vi "Continue Cycle Test.vi"(8 "error in (no error)":errorcluster, 11 "Controller in":refnum<class "Controller.lvclass">) -> (0 "error out":errorcluster, 2 "Status String":string, 3 "Controller out":refnum<class "Controller.lvclass">)   [LabVIEW 2020, in "Controller.lvlib" / "Controller.lvclass"]
uses:
  Controller.lvclass
  Controller.lvclass/Controller.ctl
  Actor_AFG/Actor_AFG Messages/AFG Wait for Complete Msg/AFG Wait for Complete Msg.lvclass/AFG Wait for Complete Msg.ctl
  <vilib>/ActorFramework/Message Enqueuer/Message Enqueuer.lvclass/Message Enqueuer.ctl
  Main_UI/Main_UI Messages/Update Cycle States Msg/Update Cycle States Msg.lvclass/Update Cycle States Msg.ctl
  <vilib>/ActorFramework/Message Enqueuer/Enqueue.vi
  Actor_AFG/Actor_AFG Messages/AFG Wait for Complete Msg/AFG Wait for Complete Msg.lvclass
  C:/Program Files/National Instruments/LabVIEW 2020/vi.lib/ActorFramework/Message/Message.lvclass
  Main_UI/Main_UI Messages/Update Cycle States Msg/Update Cycle States Msg.lvclass
  <vilib>/ActorFramework/Message Priority Queue/Priority Enqueue.vi
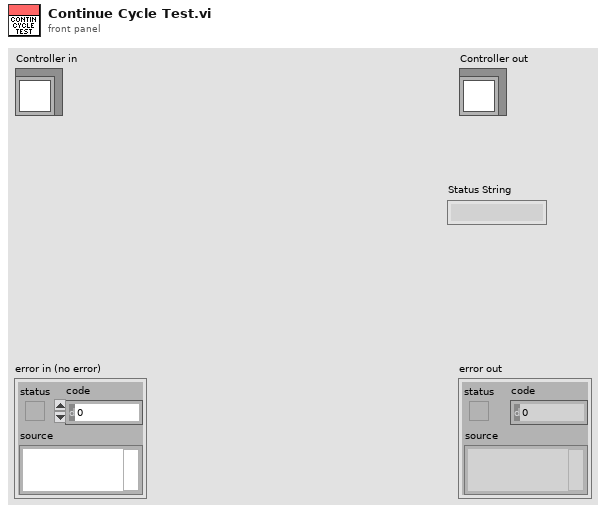
[diagram p1: front panel]
types:
  T1 = enum16{"Single Pulse", "Cycle_Idle", "Cycle_Running", "Cycle_Pause"}
  T2 = cluster{"Set Pulse Conf":cluster{"V Conf":cluster{"Bias":dbl, "Amp":dbl}, "T Conf":cluster{"Rise Time":dbl, "Fall Time":dbl, "Pulse Width":dbl}}, "Reset Pulse Conf":cluster{"V Conf":cluster{"Bias":dbl, "Amp":dbl}, "T Conf":cluster{"Rise Time":dbl, "Fall Time":dbl, "Pulse Width":dbl}}, "Cycle Timing":cluster{"Delay":dbl, "Pulse Spacing":dbl, "Burst Counts:":dbl, "Read Counts:":dbl}, "Read Voltage Setting":dbl}
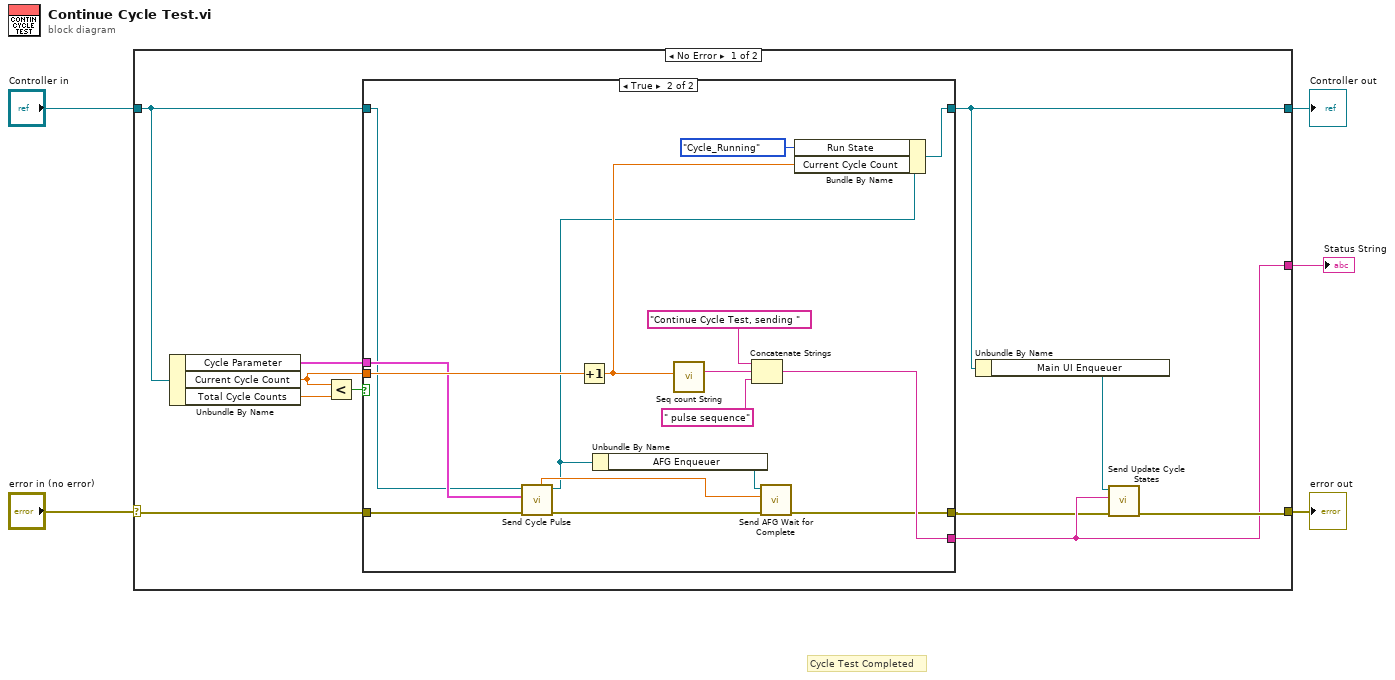
[diagram p0: block diagram]
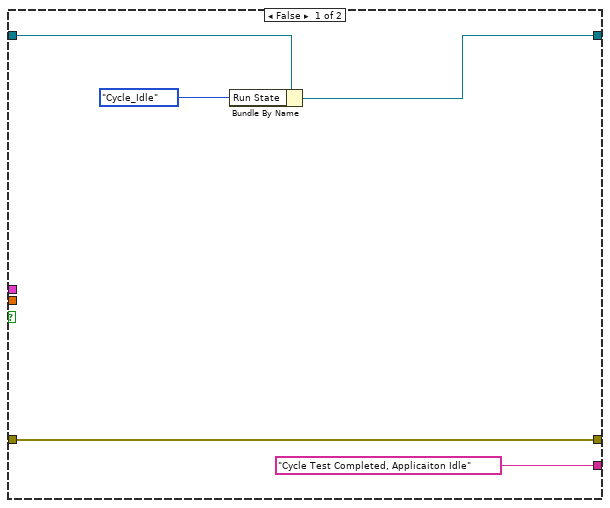
[diagram p2: hidden frame]
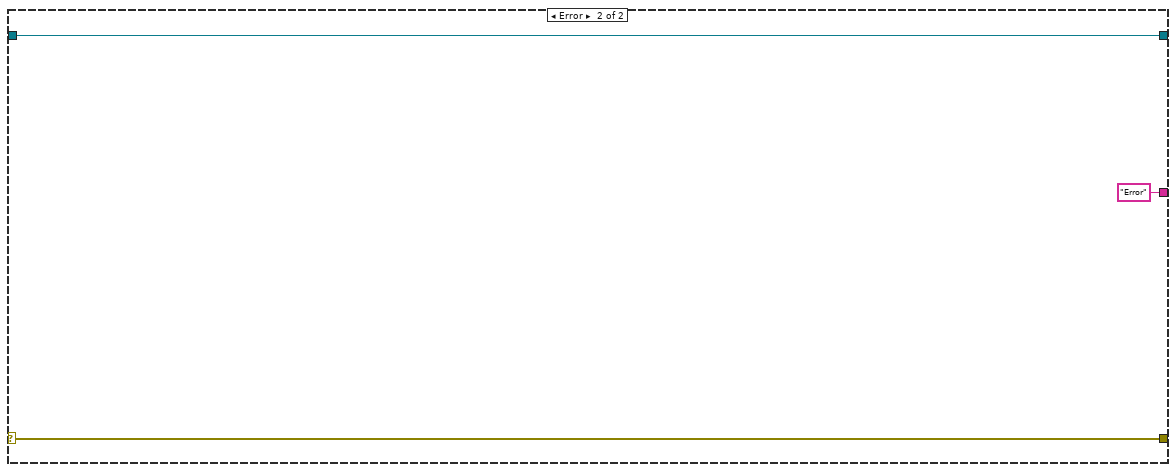
[diagram p3: hidden frame]
diagram:
  # "Cycle Test Completed"
  n1 = case shown="No Error" "error in (no error)" {
    selector: "error in (no error)" -> [w13 w40]
    tunnel: [w9 w40] -> w4
    tunnel: [w10 w39] -> w2
    tunnel: "Controller in" -> [w12 w39]
    tunnel: [w8 "Error" ("Log Event Details")] -> w1
    frame No Error {
      n2 = Unbundle By Name(w12) -> ("Cycle Parameter"=w11:T2, "Current Cycle Count"=w14:dbl, "Total Cycle Counts"=w16:dbl)
      n3 = Less?(x=w14, y=w16) -> (x < y?=w15:bool)
      n4 = case shown="True" w15 {
        tunnel: [w17 w27] -> w6
        tunnel: ["Cycle Test Completed, Applicaiton Idle" ("Log Event Details") w31] -> w8
        tunnel: w14 -> [_ w37]
        tunnel: w11 -> [_ w36]
        tunnel: w13 -> [w17 w24]
        tunnel: w12 -> [w19 w23]
        tunnel: [w18 w22] -> w10
        frame False {
          n5 = Bundle By Name(cluster=w19, "Run State"=T1."Cycle_Idle") -> (w18:refnum<class "Controller.lvclass">)
        }
        frame True {
          n6 = call "Send Cycle Pulse.vi"("error in (no error)"=w24, "Pulse Parameter"=w36, "Controller in"=w23) -> ("error out"=w29:errorcluster, "Controller Out"=w26:refnum<class "Controller.lvclass">, "Time Before OPC?"=w28:dbl)  [unwired: 4 in, 2 out]
          n7 = Increment(x=w37) -> (x+1=w35:dbl)
          n8 = Unbundle By Name(w26) -> ("AFG Enqueuer"=w25:refnum<class "Message Enqueuer.lvclass">)
          n9 = call "Seq count String.vi"("dbl in"=w35) -> ("Int String Out"=w33:string)  [unwired: 10 in]
          n10 = Concatenate Strings("Continue Cycle Test, sending ", w33, " pulse sequence") -> (w31:string)
          n11 = call "Send AFG Wait for Complete.vi"("error in (no error)"=w29, "Delay"=w28, "Message Enqueuer"=w25) -> ("error out"=w27:errorcluster)  [unwired: 7 in, 1 out]
          n12 = Bundle By Name(cluster=w26, "Run State"=T1."Cycle_Running", "Current Cycle Count"=w35) -> (w22:refnum<class "Controller.lvclass">)
        }
      }
      n13 = Unbundle By Name(w10) -> ("Main UI Enqueuer"=w7:refnum<class "Message Enqueuer.lvclass">)
      n14 = call "Send Update Cycle States.vi"("error in (no error)"=w6, "Cycle State Message"=w8, "Message Enqueuer"=w7) -> ("error out"=w9:errorcluster)  [unwired: 7 in, 1 out]
    }
    frame Error {
    }
  }
  "error out" <- w4
  "Controller out" <- w2
  "Status String" <- w1
